vi "ZCAN_Transmit(Queue).vi"(0 "can_index_handle":u32, 1 "协议":u32(ring) items=["CAN", "CANFD"], 3 "每次发送帧数（默认1）":u32=1, 5 "error in (no error)":errorcluster caption="错误输入（无错误）", 7 "ZCAN_Transmit_Data（Queue）":T2, 9 "ZCAN_TransmitFD_Data（Queue）":T1) -> (19 "error out":errorcluster caption="错误输出")   [LabVIEW 2018]
doc: "该函数用于发送CAN报文。"
uses:
  zlgcan_demo_CANFDNET_TCP/bin/zlgcan_wrap.dll
  data_type/ZCAN_Transmit_Data(Queue).ctl
  data_type/ZCAN_TransmitFD_Data(Queue).ctl
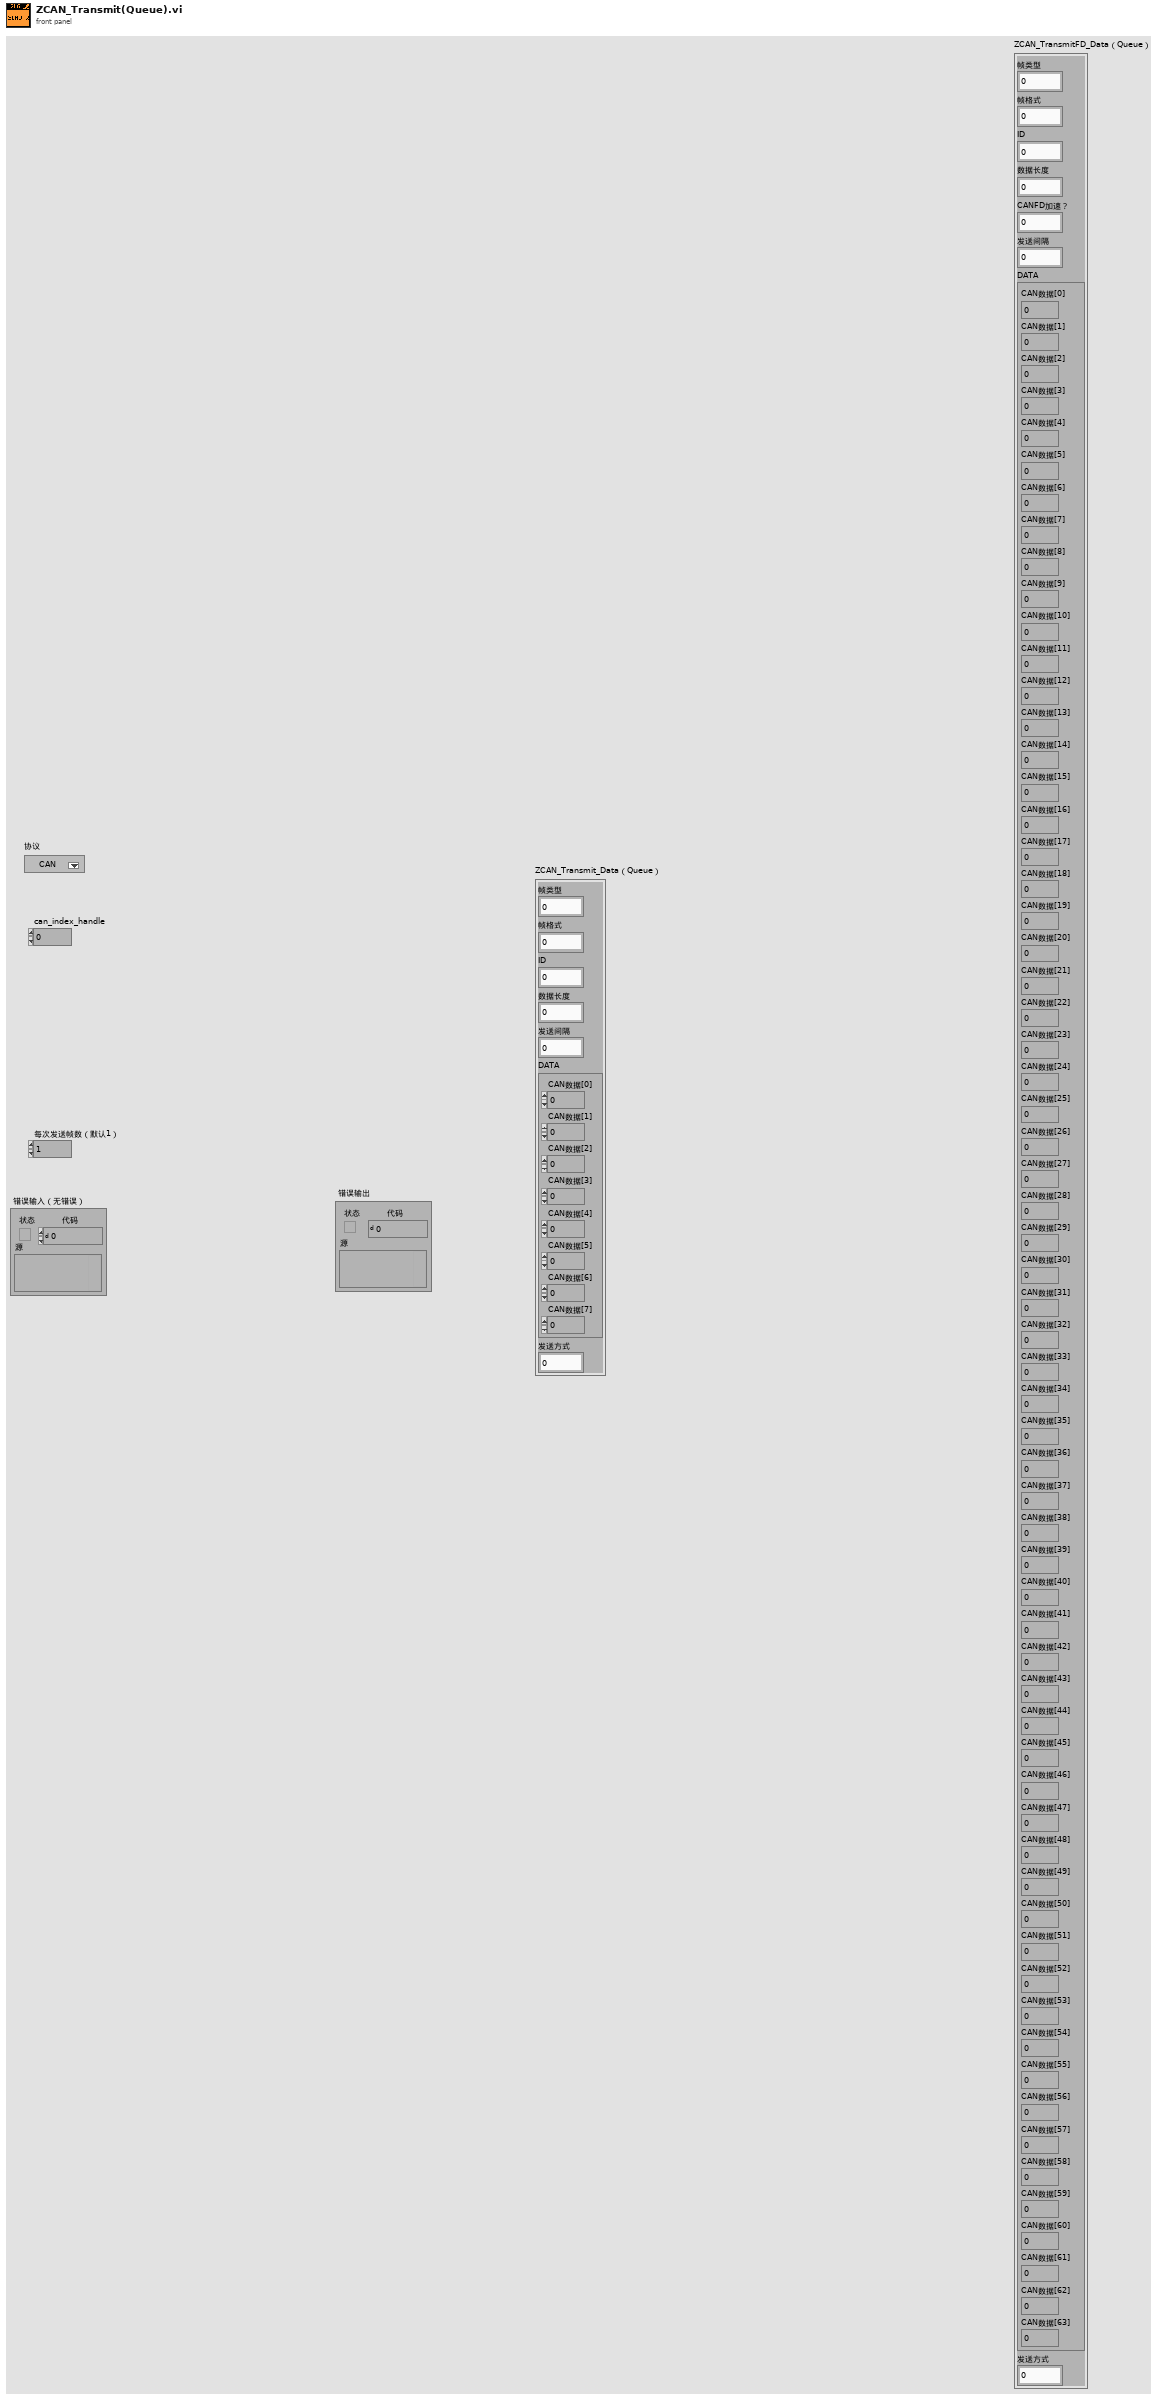
[diagram p1: front panel]
types:
  T1 = typedef "ZCAN_TransmitFD_Data(Queue).ctl" = cluster{"帧类型":u32, "帧格式":u32, "ID":u32, "数据长度":u8, "CANFD加速？":u8, "发送间隔":u16, "DATA":cluster{"CAN数据[0]":u8, "CAN数据[1]":u8, "CAN数据[2]":u8, "CAN数据[3]":u8, "CAN数据[4]":u8, "CAN数据[5]":u8, "CAN数据[6]":u8, "CAN数据[7]":u8, "CAN数据[8]":u8, "CAN数据[9]":u8, "CAN数据[10]":u8, "CAN数据[11] ":u8, "CAN数据[12] ":u8, "CAN数据[13] ":u8, "CAN数据[14] ":u8, "CAN数据[15] ":u8, "CAN数据[16]":u8, "CAN数据[17]":u8, "CAN数据[18]":u8, "CAN数据[19]":u8, "CAN数据[20]":u8, "CAN数据[21]":u8, "CAN数据[22]":u8, "CAN数据[23]":u8, "CAN数据[24] ":u8, "CAN数据[25]":u8, "CAN数据[26]":u8, "CAN数据[27]":u8, "CAN数据[28]":u8, "CAN数据[29]":u8, "CAN数据[30]":u8, "CAN数据[31]":u8, "CAN数据[32]":u8, "CAN数据[33]":u8, "CAN数据[34]":u8, "CAN数据[35]":u8, "CAN数据[36]":u8, "CAN数据[37]":u8, "CAN数据[38]":u8, "CAN数据[39]":u8, "CAN数据[40]":u8, "CAN数据[41]":u8, "CAN数据[42]":u8, "CAN数据[43]":u8, "CAN数据[44]":u8, "CAN数据[45]":u8, "CAN数据[46]":u8, "CAN数据[47]":u8, "CAN数据[48]":u8, "CAN数据[49]":u8, "CAN数据[50]":u8, "CAN数据[51]":u8, "CAN数据[52]":u8, "CAN数据[53]":u8, "CAN数据[54]":u8, "CAN数据[55]":u8, "CAN数据[56]":u8, "CAN数据[57]":u8, "CAN数据[58]":u8, "CAN数据[59]":u8, "CAN数据[60]":u8, "CAN数据[61]":u8, "CAN数据[62]":u8, "CAN数据[63]":u8}, "发送方式":u32}
  T2 = typedef "ZCAN_Transmit_Data(Queue).ctl" = cluster{"帧类型":u32, "帧格式":u32, "ID":u32, "数据长度":u8, "发送间隔":u16, "DATA":cluster{"CAN数据[0]":u8, "CAN数据[1]":u8, "CAN数据[2]":u8, "CAN数据[3]":u8, "CAN数据[4]":u8, "CAN数据[5]":u8, "CAN数据[6]":u8, "CAN数据[7]":u8}, "发送方式":u32}
  T3 = cluster{"CAN数据[0]":u8, "CAN数据[1]":u8, "CAN数据[2]":u8, "CAN数据[3]":u8, "CAN数据[4]":u8, "CAN数据[5]":u8, "CAN数据[6]":u8, "CAN数据[7]":u8, "CAN数据[8]":u8, "CAN数据[9]":u8, "CAN数据[10]":u8, "CAN数据[11] ":u8, "CAN数据[12] ":u8, "CAN数据[13] ":u8, "CAN数据[14] ":u8, "CAN数据[15] ":u8, "CAN数据[16]":u8, "CAN数据[17]":u8, "CAN数据[18]":u8, "CAN数据[19]":u8, "CAN数据[20]":u8, "CAN数据[21]":u8, "CAN数据[22]":u8, "CAN数据[23]":u8, "CAN数据[24] ":u8, "CAN数据[25]":u8, "CAN数据[26]":u8, "CAN数据[27]":u8, "CAN数据[28]":u8, "CAN数据[29]":u8, "CAN数据[30]":u8, "CAN数据[31]":u8, "CAN数据[32]":u8, "CAN数据[33]":u8, "CAN数据[34]":u8, "CAN数据[35]":u8, "CAN数据[36]":u8, "CAN数据[37]":u8, "CAN数据[38]":u8, "CAN数据[39]":u8, "CAN数据[40]":u8, "CAN数据[41]":u8, "CAN数据[42]":u8, "CAN数据[43]":u8, "CAN数据[44]":u8, "CAN数据[45]":u8, "CAN数据[46]":u8, "CAN数据[47]":u8, "CAN数据[48]":u8, "CAN数据[49]":u8, "CAN数据[50]":u8, "CAN数据[51]":u8, "CAN数据[52]":u8, "CAN数据[53]":u8, "CAN数据[54]":u8, "CAN数据[55]":u8, "CAN数据[56]":u8, "CAN数据[57]":u8, "CAN数据[58]":u8, "CAN数据[59]":u8, "CAN数据[60]":u8, "CAN数据[61]":u8, "CAN数据[62]":u8, "CAN数据[63]":u8}
  T4 = cluster{u32, "数据长度":u8, "CANFD加速？":u8, "低8位":u8, "高8位":u8, "发送方式":u32, "DATA":cluster{"CAN数据[0]":u8, "CAN数据[1]":u8, "CAN数据[2]":u8, "CAN数据[3]":u8, "CAN数据[4]":u8, "CAN数据[5]":u8, "CAN数据[6]":u8, "CAN数据[7]":u8, "CAN数据[8]":u8, "CAN数据[9]":u8, "CAN数据[10]":u8, "CAN数据[11] ":u8, "CAN数据[12] ":u8, "CAN数据[13] ":u8, "CAN数据[14] ":u8, "CAN数据[15] ":u8, "CAN数据[16]":u8, "CAN数据[17]":u8, "CAN数据[18]":u8, "CAN数据[19]":u8, "CAN数据[20]":u8, "CAN数据[21]":u8, "CAN数据[22]":u8, "CAN数据[23]":u8, "CAN数据[24] ":u8, "CAN数据[25]":u8, "CAN数据[26]":u8, "CAN数据[27]":u8, "CAN数据[28]":u8, "CAN数据[29]":u8, "CAN数据[30]":u8, "CAN数据[31]":u8, "CAN数据[32]":u8, "CAN数据[33]":u8, "CAN数据[34]":u8, "CAN数据[35]":u8, "CAN数据[36]":u8, "CAN数据[37]":u8, "CAN数据[38]":u8, "CAN数据[39]":u8, "CAN数据[40]":u8, "CAN数据[41]":u8, "CAN数据[42]":u8, "CAN数据[43]":u8, "CAN数据[44]":u8, "CAN数据[45]":u8, "CAN数据[46]":u8, "CAN数据[47]":u8, "CAN数据[48]":u8, "CAN数据[49]":u8, "CAN数据[50]":u8, "CAN数据[51]":u8, "CAN数据[52]":u8, "CAN数据[53]":u8, "CAN数据[54]":u8, "CAN数据[55]":u8, "CAN数据[56]":u8, "CAN数据[57]":u8, "CAN数据[58]":u8, "CAN数据[59]":u8, "CAN数据[60]":u8, "CAN数据[61]":u8, "CAN数据[62]":u8, "CAN数据[63]":u8}}
  T5 = cluster{u32, "数据长度":u8, "CANFD加速？":u8, "低8位":u8, "高8位":u8, "发送方式":u32, "DATA":cluster{"CAN数据[0]":u8, "CAN数据[1]":u8, "CAN数据[2]":u8, "CAN数据[3]":u8, "CAN数据[4]":u8, "CAN数据[5]":u8, "CAN数据[6]":u8, "CAN数据[7]":u8, "CAN数据[8]":u8, "CAN数据[9]":u8, "CAN数据[10]":u8, "CAN数据[11] ":u8, "CAN数据[12] ":u8, "CAN数据[13] ":u8, "CAN数据[14] ":u8, "CAN数据[15] ":u8, "CAN数据[16]":u8, "CAN数据[17]":u8, "CAN数据[18]":u8, "CAN数据[19]":u8, "CAN数据[20]":u8, "CAN数据[21]":u8, "CAN数据[22]":u8, "CAN数据[23]":u8, "CAN数据[24] ":u8, "CAN数据[25]":u8, "CAN数据[26]":u8, "CAN数据[27]":u8, "CAN数据[28]":u8, "CAN数据[29]":u8, "CAN数据[30]":u8, "CAN数据[31]":u8, "CAN数据[32]":u8, "CAN数据[33]":u8, "CAN数据[34]":u8, "CAN数据[35]":u8, "CAN数据[36]":u8, "CAN数据[37]":u8, "CAN数据[38]":u8, "CAN数据[39]":u8, "CAN数据[40]":u8, "CAN数据[41]":u8, "CAN数据[42]":u8, "CAN数据[43]":u8, "CAN数据[44]":u8, "CAN数据[45]":u8, "CAN数据[46]":u8, "CAN数据[47]":u8, "CAN数据[48]":u8, "CAN数据[49]":u8, "CAN数据[50]":u8, "CAN数据[51]":u8, "CAN数据[52]":u8, "CAN数据[53]":u8, "CAN数据[54]":u8, "CAN数据[55]":u8, "CAN数据[56]":u8, "CAN数据[57]":u8, "CAN数据[58]":u8, "CAN数据[59]":u8, "CAN数据[60]":u8, "CAN数据[61]":u8, "CAN数据[62]":u8, "CAN数据[63]":u8}}[]
  T6 = cluster{"CAN数据[0]":u8, "CAN数据[1]":u8, "CAN数据[2]":u8, "CAN数据[3]":u8, "CAN数据[4]":u8, "CAN数据[5]":u8, "CAN数据[6]":u8, "CAN数据[7]":u8}
  T7 = cluster{u32, "数据长度":u8, u8, "低8位":u8, "高8位":u8, "DATA":cluster{"CAN数据[0]":u8, "CAN数据[1]":u8, "CAN数据[2]":u8, "CAN数据[3]":u8, "CAN数据[4]":u8, "CAN数据[5]":u8, "CAN数据[6]":u8, "CAN数据[7]":u8}, "发送方式":u32}
  T8 = cluster{u32, "数据长度":u8, u8, "低8位":u8, "高8位":u8, "DATA":cluster{"CAN数据[0]":u8, "CAN数据[1]":u8, "CAN数据[2]":u8, "CAN数据[3]":u8, "CAN数据[4]":u8, "CAN数据[5]":u8, "CAN数据[6]":u8, "CAN数据[7]":u8}, "发送方式":u32}[]
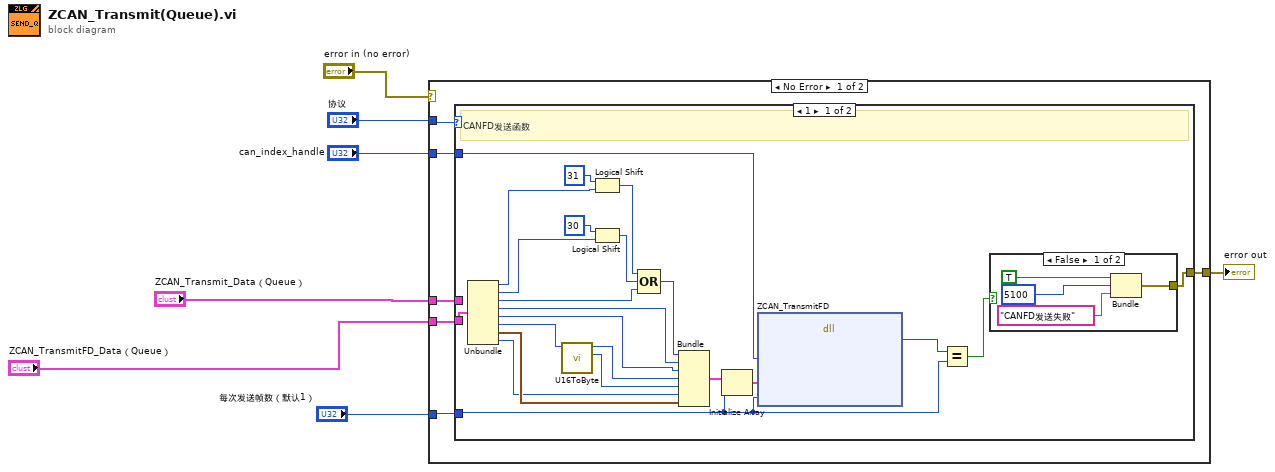
[diagram p0: block diagram]
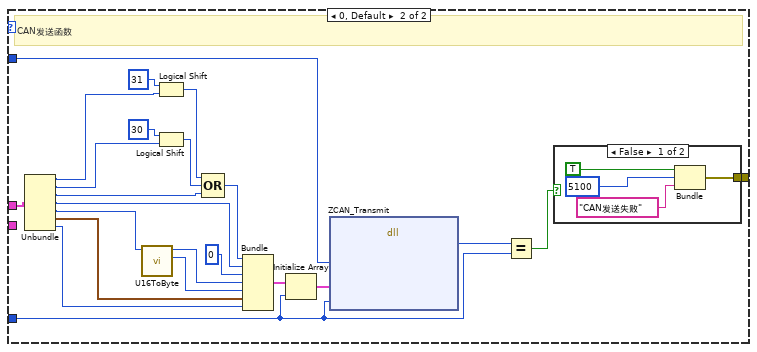
[diagram p3: hidden frame]
diagram:
  n1 = case shown="No Error" "error in (no error)" {
    selector: "error in (no error)" -> [_ w68]
    tunnel: [w13 w68] -> w6
    tunnel: "每次发送帧数（默认1）" -> [w12 _]
    tunnel: "can_index_handle" -> [w11 _]
    tunnel: "协议" -> [w10 _]
    tunnel: "ZCAN_Transmit_Data（Queue）" -> [w9 _]
    tunnel: "ZCAN_TransmitFD_Data（Queue）" -> [w8 _]
    frame No Error {
      n2 = case shown="1" w10 {
        tunnel: [w18 w55] -> w13
        tunnel: w12 -> [w19 w54]
        tunnel: w11 -> [w23 w51]
        tunnel: w9 -> [_ w48]
        tunnel: w8 -> [w22 _]
        frame 1 {
          # "CANFD发送函数"
          n3 = Unbundle(w22) -> ("帧类型"=w27:u32, "帧格式"=w26:u32, "ID"=w25:u32, "数据长度"=w24:u8, "CANFD加速？"=w21:u8, "发送间隔"=w16:u16, "DATA"=w20:T3, "发送方式"=w17:u32)
          n4 = call "U16ToByte.vi"("数值"=w16) -> ("高8位"=w14:u8, "低8位"=w15:u8)  [unwired: 9 in]
          n5 = Logical Shift(y=i16 31, x=w27) -> (x << y=w34:u32)
          n6 = Logical Shift(y=i16 30, x=w26) -> (x << y=w31:u32)
          n7 = Compound Arithmetic op=OR ("复合运算")(w34, w31, w25) -> (w30:u32)
          n8 = Bundle ("捆绑")(w30, "数据长度"=w24, "CANFD加速？"=w21, "低8位"=w15, "高8位"=w14, "发送方式"=w17, "DATA"=w20) -> (w36:T4)  [unwired: 1 in]
          n9 = Initialize Array(w36, w19) -> (w35:T5)
          n10 = dll-call lib="C:/Users/admin/Desktop/zlgcan_demo_CANFDNET_TCP/bin/zlgcan_wrap.dll" fn="ZCAN_TransmitFD"("通道句柄"=w23, "数据帧数组"=w35, "数据帧数"=w19) -> ("返回类型"=w29:u32)  [unwired: 6 in, 2 out]
          n11 = Equal?(x=w29, y=w19) -> (x = y?=w28:bool)
          n12 = case shown="False" w28 {
            tunnel: [w37 _] -> w18
            frame False {
              n13 = Bundle("status"=TRUE, "code"=5100, "消息"="CANFD发送失败") -> (w37:cluster{"status":bool, "code":i32, "消息":string})  [unwired: 1 in]
            }
            frame True {
            }
          }
        }
        frame 0, Default {
          # "CAN发送函数"
          n14 = Unbundle(w48) -> ("帧类型"=w41:u32, "帧格式"=w42:u32, "ID"=w43:u32, "数据长度"=w44:u8, "发送间隔"=w45:u16, "DATA"=w46:T6, "发送方式"=w47:u32)
          n15 = call "U16ToByte.vi"("数值"=w45) -> ("高8位"=w49:u8, "低8位"=w50:u8)  [unwired: 9 in]
          n16 = Logical Shift(y=i16 31, x=w41) -> (x << y=w60:u32)
          n17 = Logical Shift(y=i16 30, x=w42) -> (x << y=w57:u32)
          n18 = Compound Arithmetic op=OR ("复合运算")(w60, w57, w43) -> (w56:u32)
          n19 = Bundle ("捆绑")(w56, "数据长度"=w44, u8 0, "低8位"=w50, "高8位"=w49, "DATA"=w46, "发送方式"=w47) -> (w62:T7)  [unwired: 1 in]
          n20 = Initialize Array(w62, w54) -> (w61:T8)
          n21 = dll-call lib="C:/Users/admin/Desktop/zlgcan_demo_CANFDNET_TCP/bin/zlgcan_wrap.dll" fn="ZCAN_Transmit"("通道句柄"=w51, "数据帧数组"=w61, "数据帧数"=w54) -> ("返回类型"=w53:u32)  [unwired: 6 in, 2 out]
          n22 = Equal?(x=w53, y=w54) -> (x = y?=w52:bool)
          n23 = case shown="False" w52 {
            tunnel: [w64 _] -> w55
            frame False {
              n24 = Bundle("status"=TRUE, "code"=5100, "消息"="CAN发送失败") -> (w64:cluster{"status":bool, "code":i32, "消息":string})  [unwired: 1 in]
            }
            frame True {
            }
          }
        }
      }
    }
    frame Error {
    }
  }
  "error out" <- w6
